vi "uActor_Get Self Transport.vi"(11 "uActor in":refnum<class "uActor.lvclass">) -> (2 "Actor Transport":refnum<class "uTransport_uActor.lvclass">, 3 "uActor out":refnum<class "uActor.lvclass">)   [LabVIEW 2023, in "uLib.lvlib" / "uActor.lvclass"]
uses:
  uActor.lvclass
  uTransport/uTransport_uActor/uTransport_uActor.lvclass
  uActor.lvclass/uActor.ctl
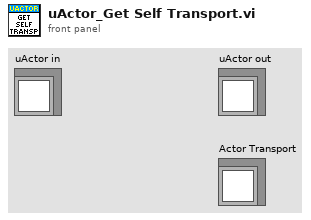
[diagram p1: front panel]
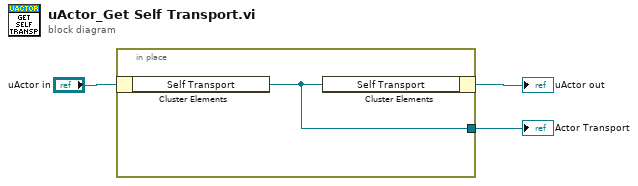
[diagram p0: block diagram]
diagram:
  n1 = in-place {
    in-place-border: [w4] -> w1
    n2 = in-place-cluster #1("uActor in") -> ("Self Transport"=w4:refnum<class "uTransport_uActor.lvclass">)
    n3 = in-place-cluster #1("Self Transport"=w4) -> (→"uActor out":refnum<class "uActor.lvclass">)
  }
  "Actor Transport" <- w1
